vi "Loop_ACT_Elbow.vi"() -> ()   [LabVIEW 2017, in "Lift.lvlib"]
uses:
  Lift.lvlib
  _SHARE ALL/TypeDef Share All/CLUSTER_TalonOutput.ctl
  _SHARE ALL/TypeDef Share All/CLUSTER_TalonInput.ctl
  System Drivers/Phoenix-LabVIEW/Motor Controller/Controls/CTRE_Phoenix_MotorControl_ControlMode.ctl
  _SHARE ALL/RoboRio Share All/SRX Share All/TypeDefs SRX/Cluster_SRX_PIDF.ctl
  _SHARE ALL/TypeDef Share All/CONTROL_PositonGraph.ctl
  TypeDef/CLUSTER_PID.ctl
  CLUSTER_ACT_Lift Output.ctl
  _SHARE ALL/RoboRio Share All/SRX Share All/TypeDefs SRX/Cluster_SRX_General Data.ctl
  _SHARE ALL/RoboRio Share All/SRX Share All/TypeDefs SRX/Cluster_SRX_Common Runtime Data.ctl
  _SHARE ALL/RoboRio Share All/SRX Share All/TypeDefs SRX/Cluster_SRX_Error Calculations.ctl
  _SHARE ALL/RoboRio Share All/SRX Share All/TypeDefs SRX/Cluster_SRX_Voltage Out Data.ctl
  _SHARE ALL/RoboRio Share All/SRX Share All/TypeDefs SRX/Cluster_SRX_Sensor Out Data.ctl
  _SHARE ALL/RoboRio Share All/SRX Share All/TypeDefs SRX/Cluster_SRX_Sensor Quad Data.ctl
  _SHARE ALL/RoboRio Share All/SRX Share All/TypeDefs SRX/Cluster_SRX_Analog In Data.ctl
  _SHARE ALL/RoboRio Share All/SRX Share All/TypeDefs SRX/Cluster_SRX_PWM Sensor Data.ctl
  _SHARE ALL/RoboRio Share All/SRX Share All/TypeDefs SRX/Cluster_SRX_F and R Limit Indicators.ctl
  Globals/Global_Device_IDs.vi
  _SHARE ALL/Global Share All/Global_STOP.vi
  Global_SM Write_Data Out.vi
  System Drivers/Phoenix-LabVIEW/Motor Controller/Get/CTRE_Phoenix_MotorController_GetSelectedSensorData.vi
  System Drivers/Phoenix-LabVIEW/Motor Controller/Get/CTRE_Phoenix_MotorController_GetVoltage.vi
  Global_ACT Write_Data Out.vi
panel:
  in  "Display Graph":bool
  out "Position Closed Loop Plots":T1
  out "Elbow Input":T2 {"Talon Mode" items=["PercentOutput"=0, "Position"=1, "Velocity"=2, "Current"=3, "Follower"=5, "MotionProfile"=6, "MotionMagic"=7, "MotionMagicArc"=8, "MotionProfileArc"=10, "Disabled"=15]}
  out "Elbow Output":T5
  out "Cycle Time (S)":dbl format="%.3g"
  in  "Target Time(ms)":u32=50
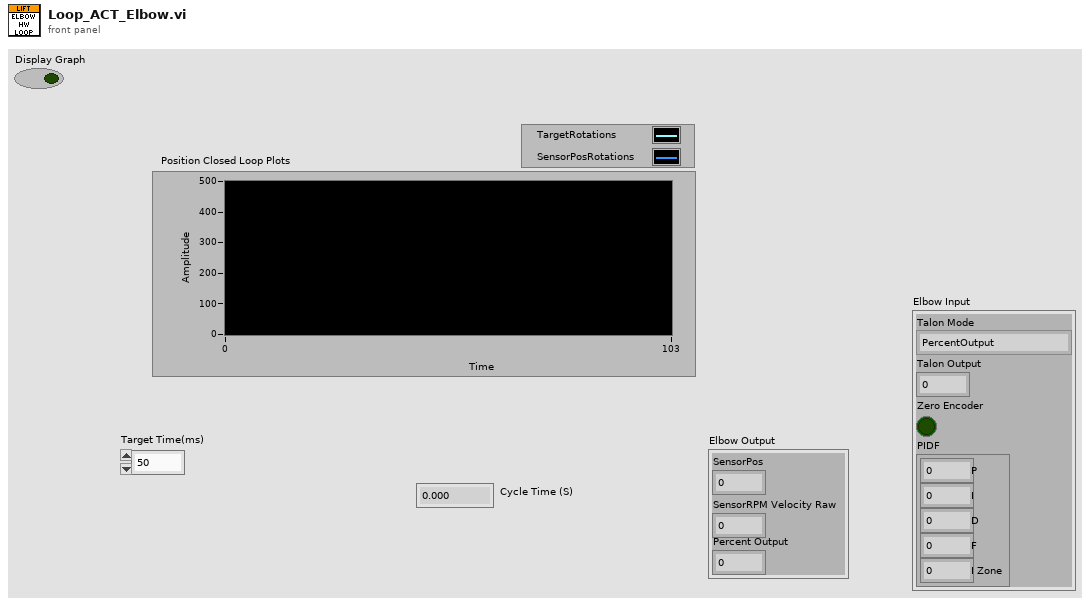
[diagram p1: front panel]
types:
  T1 = typedef "CONTROL_PositonGraph.ctl" = cluster{dbl, "Position (Raw Sensor Units)":i32}
  T2 = typedef "CLUSTER_TalonInput.ctl" = cluster{"Talon Mode":T3, "Talon Output":dbl, "Zero Encoder":bool, "PIDF":T4}
  T3 = typedef "CTRE_Phoenix_MotorControl_ControlMode.ctl" = u16
  T4 = typedef "Cluster_SRX_PIDF.ctl" = cluster{"P":dbl, "I":dbl, "D":dbl, "F":dbl, "I Zone":dbl}
  T5 = typedef "CLUSTER_TalonOutput.ctl" = cluster{"SensorPos":i32, "SensorRPM Velocity Raw":i32, "Percent Output":dbl}
  T6 = typedef "Lift.lvlib/CLUSTER_ACT_Lift Output.ctl" = cluster{"Device Info Out":T7, "Common Runtime Data Out":T8, "Quad Sensor Data Out":T12, "Analog Sensor Data Out":T13, "PWM Data Out":T14, "Hard Limits Out":T15}
  T7 = typedef "Cluster_SRX_General Data.ctl" = cluster{"Device ID":i32, "Firmware Version":i32, "Inverted?":bool, "Has Reset Occurred?":bool}
  T8 = typedef "Cluster_SRX_Common Runtime Data.ctl" = cluster{"Calc":T9, "Voltage ":T10, "Sensor":T11, "Current":dbl, "Temp":dbl}
  T9 = typedef "Cluster_SRX_Error Calculations.ctl" = cluster{"Error":i32, "D-Error":dbl, "I-Acc":dbl}
  T10 = typedef "Cluster_SRX_Voltage Out Data.ctl" = cluster{"Percent":dbl, "Output":dbl, "Bus":dbl}
  T11 = typedef "Cluster_SRX_Sensor Out Data.ctl" = cluster{"Pos":i32, "Vel":i32}
  T12 = typedef "Cluster_SRX_Sensor Quad Data.ctl" = cluster{"Position":i32, "Velocity":i32, "Quad A Pin":bool, "Quad B Pin":bool, "Quad Idx Pin":bool}
  T13 = typedef "Cluster_SRX_Analog In Data.ctl" = cluster{"WithOv":i32, "Raw":i32, "Velocity":i32}
  T14 = typedef "Cluster_SRX_PWM Sensor Data.ctl" = cluster{"Position":i32, "Velocity":i32, "High(us)":i32, "Period(us)":i32}
  T15 = typedef "Cluster_SRX_F and R Limit Indicators.ctl" = cluster{"Forward Closed?":bool, "Reverse Closed?":bool}
  T16 = typedef "CLUSTER_PID.ctl" = cluster{"P":dbl, "I":dbl, "D":dbl, "F":dbl, "I Zone":dbl}
  T17 = typedef "CLUSTER_Arm_Device_IDs.ctl" = cluster{"Elbow Setup":T18, "Telescope Setup":T18, "Elbow Slave Setup":T18, "Telescope Slave Setup":T18}
  T18 = typedef "CLUSTER_Talon_Setup.ctl" = cluster{"Talon SRX ID":u8, "PhaseSensor":bool, "Invert Motor?":bool, "Phoenix Feedback Select":T19, "pidLoopldx":i32, "PID":T16}
  T19 = typedef "CTRE_Phoenix_MotorControl_FeedbackDevice.ctl" = i8
  T20 = typedef "WPI_MotorControlDeviceRef.ctl" = cluster{"DeviceStatus":errorcluster, "Type":T21, "PWM":cluster{"PWM Channel":T22, "DeadBand":T23}, "CAN":cluster{"Device Number":u8, "SetOutput VI Ref":variant, "GetOutput VI Ref":variant, "Enable VI Ref":variant, "Disable VI Ref":variant, "Data":variant}, "Invert":bool, "DIO PWM":cluster{"PWM \"Enable\" Channel":T22, "DIOChannel":T24, "PWM Rate":dbl}}
  T21 = typedef "WPI_MotorControlType.ctl" = enum16{"PWM", "CAN", "DIO PWM"}
  T22 = typedef "FPGA_DIOPWMChannel.ctl" = enum8{"PWM 0", "PWM 1", "PWM 2", "PWM 3", "PWM 4", "PWM 5", "PWM 6", "PWM 7", "PWM 8", "PWM 9", "PWM MXP 0", "PWM MXP 1", "PWM MXP 2", "PWM MXP 3", "PWM MXP 4", "PWM MXP 5", "PWM MXP 6", "PWM MXP 7", "PWM MXP 8", "PWM MXP 9", "Invalid"}
  T23 = typedef "WPI_PWMDeadband.ctl" = cluster{"Name":string, "maxPositivePwm":i32, "minPositivePwm":i32, "centerPwm":i32, "maxNegativePwm":i32, "minNegativePwm":i32, "angularRange":u16}
  T24 = typedef "FPGA_DIOChannel.ctl" = enum8{"DIO 0", "DIO 1", "DIO 2", "DIO 3", "DIO 4", "DIO 5", "DIO 6", "DIO 7", "DIO 8", "DIO 9", "DIO MXP 0", "DIO MXP 1", "DIO MXP 2", "DIO MXP 3", "DIO MXP 4", "DIO MXP 5", "DIO MXP 6", "DIO MXP 7", "DIO MXP 8", "DIO MXP 9", "DIO MXP 10", "DIO MXP 11", "DIO MXP 12", "DIO MXP 13", "DIO MXP 14", "DIO MXP 15", "SPI Port CS1", "SPI Port CS2", "SPI Port CS3", "SPI Port MISO", "SPI Port MOSI", "Invalid"}
  T25 = cluster{"PhoenixMotorControlDevRef":T20, "Elbow Output":T5, "Elbow Input":T2, "Target Time(ms)":u32, "Current Time":timestamp, "Previous Time":timestamp, "Cycle Time (S)":dbl, "Last PID":T16}
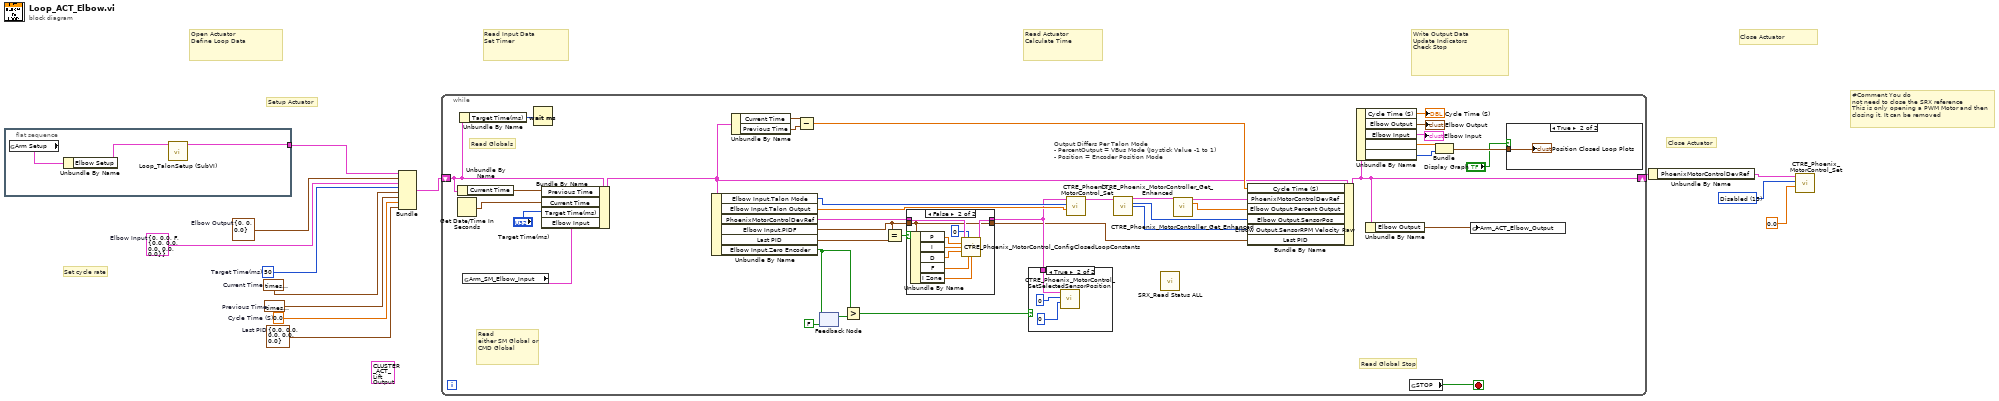
[diagram p0: block diagram]
diagram:
  (unwired) T6 {"Device Info Out"={"Device ID"=0, "Firmware Version"=0, "Inverted?"=FALSE, "Has Reset Occurred?"=FALSE}, "Common Runtime Data Out"={"Calc"={"Error"=0, "D-Error"=0.0, "I-Acc"=0.0}, "Voltage "={"Percent"=0.0, "Output"=0.0, "Bus"=0.0}, "Sensor"={"Pos"=0, "Vel"=0}, "Current"=0.0, "Temp"=0.0}, "Quad Sensor Data Out"={"Position"=0, "Velocity"=0, "Quad A Pin"=FALSE, "Quad B Pin"=FALSE, "Quad Idx Pin"=FALSE}, "Analog Sensor Data Out"={"WithOv"=0, "Raw"=0, "Velocity"=0}, "PWM Data Out"={"Position"=0, "Velocity"=0, "High(us)"=0, "Period(us)"=0}, "Hard Limits Out"={"Forward Closed?"=FALSE, "Reverse Closed?"=FALSE}}
  w2 = T16 {"P"=0.0, "I"=0.0, "D"=0.0, "F"=0.0, "I Zone"=0.0}  # Last PID
  w4 = T3 15 items=["PercentOutput"=0, "Position"=1, "Velocity"=2, "Current"=3, "Follower"=5, "MotionProfile"=6, "MotionMagic"=7, "MotionMagicArc"=8, "MotionProfileArc"=10, "Disabled"=15] ("Control Mode")
  w6 = T5 {"SensorPos"=0, "SensorRPM Velocity Raw"=0, "Percent Output"=0.0}  # Elbow Output
  w7 = T2 {"Talon Mode"=0, "Talon Output"=0.0, "Zero Encoder"=FALSE, "PIDF"={"P"=0.0, "I"=0.0, "D"=0.0, "F"=0.0, "I Zone"=0.0}}  # Elbow Input
  w8 = 0.0  # Cycle Time (S)
  w13 = timestamp(0 s since 1904-01-01)  # Previous Time
  w12 = timestamp(0 s since 1904-01-01)  # Current Time
  w11 = u32 50  # Target Time(ms)
  # "#Comment You do\nnot need to close the SRX reference\nThis is only opening a PWM Motor and then\nclosing it. It can be removed"
  # "Close Actuator"
  # "Write Output Data\nUpdate Indicators\nCheck Stop"
  # "Read Actuator\nCalculate Time"
  # "Read Input Data\nSet Timer"
  # "Open Actuator\nDefine Loop Data"
  # "Set cycle rate"
  # "Close Actuator"
  # "Setup Actuator"
  n1 = flat-sequence {
    tunnel: [w14] -> w1
    frame #0 {
      n2 = global read "Global_Device_IDs.vi" "Arm Setup"() -> (w16:T17)
      n3 = Unbundle By Name(w16) -> ("Elbow Setup"=w15:T18)
      n4 = call "Loop_TalonSetup (SubVI).vi"("Elbow Setup"=w15) -> ("PhoenixMotorControlDevRef"=w14:T20)  [unwired: 10 in]
    }
  }
  n5 = Bundle("PhoenixMotorControlDevRef"=w1, "Elbow Output"=w6, "Elbow Input"=w7, "Target Time(ms)"=w11, "Current Time"=w12, "Previous Time"=w13, "Cycle Time (S)"=w8, "Last PID"=w2) -> (w10:T25)  [unwired: 1 in]
  n6 = while {
    shift-right: [w46] -> w9
    shift-left: w10 -> [w48]
    stop <- w54 stop-if-true
    # "Output Differs Per Talon Mode\n- PercentOutput = VBus Mode (Joystick Value -1 to 1)\n- Position = Encoder Position Mode"
    # "Read\neither SM Global or CMD Global"
    # "Read Globals"
    # "Read Global Stop"
    n7 = Unbundle By Name(w48) -> ("Current Time"=w52:timestamp)
    n8 = Get Date/Time In Seconds() -> (seconds since 1Jan1904=w53:timestamp)
    n9 = Unbundle By Name(w48) -> ("Target Time(ms)"=w47:u32)
    n10 = global read "Global_SM Write_Data Out.vi" "Arm_SM_Elbow_Input"() -> (w42:T2)
    n11 = Wait (ms)(milliseconds to wait=w47) -> ()  [unwired: 1 out]
    n12 = Bundle By Name(cluster=w48, "Previous Time"=w52, "Current Time"=w53, "Target Time(ms)"="Target Time(ms)", "Elbow Input"=w42) -> (w31:T25)
    n13 = Unbundle By Name(w31) -> ("Elbow Input.Talon Mode"=w41:T3, "Elbow Input.Talon Output"=w40:dbl, "PhoenixMotorControlDevRef"=w30:T20, "Elbow Input.PIDF"=w26:T4, "Last PID"=w27:T16, "Elbow Input.Zero Encoder"=w22:bool)
    n14 = Unbundle By Name(w31) -> ("Current Time"=w51:timestamp, "Previous Time"=w50:timestamp)
    n15 = Subtract(x=w51, y=w50) -> (x-y=w44:dbl)
    n16 = feedback #1(FALSE) -> (w23:bool)
    n17 = feedback-in #1(w22) -> ()
    n18 = Greater?(x=w22, y=w23) -> (0:w21:bool)
    n19 = Equal?(x=w26, y=w27) -> (x = y?=w25:bool)
    n20 = case shown="False" w25 {
      tunnel: w30 -> [w56 w65]
      tunnel: [w56 w64] -> w29
      tunnel: w26 -> [w55 w57]
      tunnel: [w55 w57] -> w17
      frame True {
      }
      frame False {
        n21 = Unbundle By Name(w57) -> ("P"=w62:dbl, "I"=w61:dbl, "D"=w60:dbl, "F"=w59:dbl, "I Zone"=w58:dbl)
        n22 = call "CTRE_Phoenix_MotorControl_ConfigClosedLoopConstants.vi"("PhoenixMotorControlDevRef"=w65, "slotIdx"=0, "P"=w62, "I"=w61, "D"=w60, "F"=w59, "I Zone"=w58) -> ("PhoenixMotorControlDevRef"=w64:T20)  [unwired: 7 in, 1 out]
      }
    }
    n23 = case shown="True" w21 {
      tunnel: w29 -> [_ w69]
      frame False {
      }
      frame True {
        n24 = call "CTRE_Phoenix_MotorControl_SetSelectedSensorPosition.vi"("pidLoopIdx"=u32 0, "New Sensor Position"=0, "PhoenixMotorControlDevRef"=w69) -> ()  [unwired: 7 in, 2 out]
      }
    }
    n25 = call "CTRE_Phoenix_MotorControl_Set.vi"("Output"=w40, "Control Mode"=w41, "PhoenixMotorControlDevRef"=w29) -> ("PhoenixMotorControlDevRef"=w39:T20)  [unwired: 7 in, 1 out]
    n26 = call-poly "CTRE_Phoenix_MotorController_Get_Enhanced.vi"("PhoenixMotorControlDevRef"=w39) -> ("PhoenixMotorControlDevRef"=w38:T20, "Position (Raw Sensor Units)"=w19:i32, "Velocity (Raw Sensor Units per 100 ms)"=w18:i32)  [unwired: 11 in, 1 out]
    n27 = call "SRX_Read Status ALL.vi"() -> ()  [unwired: 5 in, 7 out]
    n28 = call-poly "CTRE_Phoenix_MotorController_Get_Enhanced.vi"("PhoenixMotorControlDevRef"=w38) -> ("PhoenixMotorControlDevRef"=w20:T20, "Percent Output"=w37:dbl)  [unwired: 10 in, 3 out]
    n29 = Bundle By Name(cluster=w31, "Cycle Time (S)"=w44, "PhoenixMotorControlDevRef"=w20, "Elbow Output.Percent Output"=w37, "Elbow Output.SensorPos"=w19, "Elbow Output.SensorRPM Velocity Raw"=w18, "Last PID"=w17) -> (w46:T25)
    n30 = Unbundle By Name(w46) -> ("Cycle Time (S)"=→"Cycle Time (S)":dbl, "Elbow Output"=→"Elbow Output":T5, "Elbow Input"=→"Elbow Input":T2, "Elbow Input.Talon Output"=w34:dbl, "Elbow Output.SensorPos"=w33:i32)
    n31 = Unbundle By Name(w46) -> ("Elbow Output"=w43:T5)
    n32 = global read "Global_STOP.vi" "STOP"() -> (w54:bool)
    n33 = Bundle("Talon Output"=w34, "SensorPos"=w33) -> (w32:cluster{"Talon Output":dbl, "SensorPos":i32})  [unwired: 1 in]
    n34 = global write "Global_ACT Write_Data Out.vi" "Arm_ACT_Elbow_Output"(w43) -> ()
    n35 = case shown="True" "Display Graph" {
      tunnel: w32 -> [_ w66]
      frame False {
      }
      frame True {
        "Position Closed Loop Plots" <- w66
      }
    }
  }
  n36 = Unbundle By Name(w9) -> ("PhoenixMotorControlDevRef"=w5:T20)
  n37 = call "CTRE_Phoenix_MotorControl_Set.vi"("Output"=0.0, "Control Mode"=w4, "PhoenixMotorControlDevRef"=w5) -> ()  [unwired: 7 in, 2 out]
